vi "Pre Launch Init.vi"(11 "Tcp in":refnum<class "Tcp.lvclass">) -> (0 "error out":errorcluster, 3 "Tcp out":refnum<class "Tcp.lvclass">)   [LabVIEW 2022 SP3, in "Tcp.lvlib" / "Tcp.lvclass"]
doc: "(<B>Filename</B>: Actor Framework.lvlib:Actor.lvclass:Pre Launch Init.vi)\n\nDefines behavior that occurs after the Launch Actor method is invoked but before the actor's Actor Core method begins running.\n\nThe Pre Launch Init method is guaranteed to finish before the Launch Actor method returns to its caller and before the actor itself receives any messages. Any references that the Pre Launch Init method obtains are guaranteed to have the same lifetime as the actor itself. Any errors that the Pre Launch Init method returns will abort the launch.\n\nBy default, this method does nothing. A descendant class may override it to define behavior."
uses:
  Tcp.lvclass
  Tcp.lvclass/Tcp.ctl
  TcpSocket/Source/TcpSocket/TcpServer/TcpServer.lvclass
  <vilib>/ActorFramework/Actor/Actor.lvclass
  Tcp Messages/WaitForConnection Msg/WaitForConnection Msg.lvclass
  Logger/Source/Logger/_Level.ctl
  Logger/Source/Logger/Logger.lvclass
  DateTime/Source/DateTime.lvlib
  Logger/Source/Handler/Handler.lvclass
  Logger/Source/FileHandler/FileHandler.lvclass
  C:/Users/jakub/repos/gh/lv-cli-framework/Logger/Source/Handler/Handler.lvclass
  C:/Program Files (x86)/National Instruments/LabVIEW 2022/vi.lib/ActorFramework/Actor/Actor.lvclass
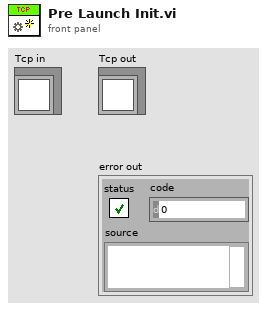
[diagram p1: front panel]
types:
  T1 = typedef "Logger.lvlib/Logger.lvclass/_Level.ctl" = enum16{"NOTSET", "DEBUG", "INFO", "WARNING", "ERROR", "CRITICAL"}
  T2 = enum16{"Standard", "Buffered", "CRLF", "Immediate"}
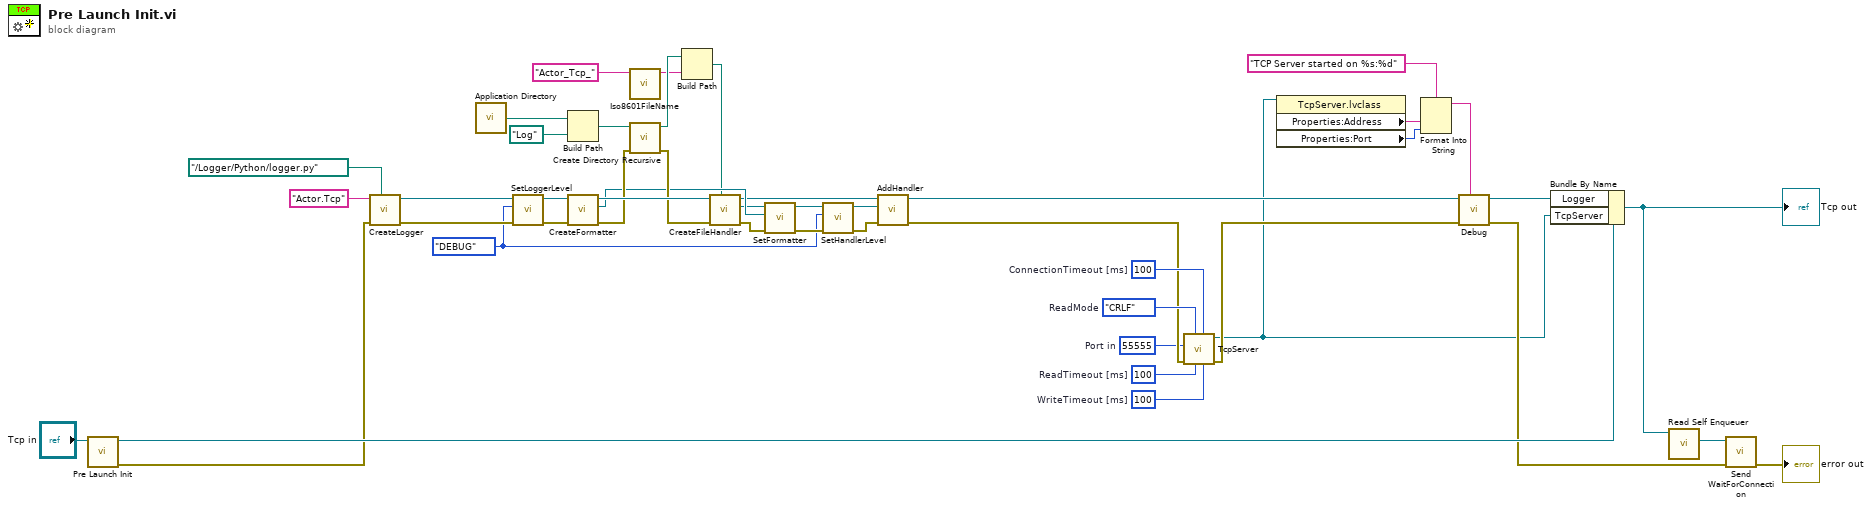
[diagram p0: block diagram]
diagram:
  w2 = _Level."DEBUG" ("Level")
  w43 = 100  # ConnectionTimeout [ms]
  w44 = 100  # WriteTimeout [ms]
  w45 = 100  # ReadTimeout [ms]
  w46 = T2."CRLF"  # ReadMode
  w16 = u16 55555  # Port in
  n1 = call-parent "Pre Launch Init.vi"("Actor in"="Tcp in") -> ("error out"=w23:errorcluster, "Actor out"=w42:refnum<class "Tcp.lvclass">)  [unwired: 9 in]
  n2 = call "CreateLogger.vi"("ModulePath"=path "../Logger/Python/logger.py" ("name or relative path"), "error in (no error)"=w23, "Name"="Actor.Tcp") -> ("error out"=w38:errorcluster, "Logger"=w37:refnum<class "Logger.lvclass">)  [unwired: 7 in]
  n3 = call <vilib>:"Application Directory.vi"() -> ("Application Directory"=w9:path)
  n4 = call-dynamic "SetLoggerLevel.vi"("error in (no error)"=w38, "Level"=w2, "Logger in"=w37) -> ("error out"=w35:errorcluster, "Logger out"=w36:refnum<class "Logger.lvclass">)  [unwired: 7 in]
  n5 = Build Path(base path=w9, name or relative path=path "Log") -> (appended path=w7:path)
  n6 = call-dynamic "CreateFormatter.vi"("error in (no error)"=w35, "Logger in"=w36) -> ("error out"=w32:errorcluster, "Formatter"=w28:refnum<class "Formatter.lvclass">, "Logger out"=w34:refnum<class "Logger.lvclass">)  [unwired: 7 in]
  n7 = call "Iso8601FileName.vi"("Prefix ('')"="Actor_Tcp_") -> ("FileName"=w5:string)  [unwired: 10 in]
  n8 = call <vilib>:"Create Directory Recursive.vi"("error in (no error)"=w32, "directory"=w7) -> ("error out"=w31:errorcluster, "directory copy"=w6:path)  [unwired: 3 in, 1 out]
  n9 = Build Path(base path=w6, name or relative path=w5) -> (appended path=w4:path)
  n10 = call-dynamic "CreateFileHandler.vi"("FIlePath"=w4, "error in (no error)"=w31, "Logger in"=w34) -> ("error out"=w30:errorcluster, "FileHandler"=w27:refnum<class "FileHandler.lvclass">, "Logger out"=w3:refnum<class "Logger.lvclass">)  [unwired: 6 in]
  n11 = call "SetFormatter.vi"("error in (no error)"=w30, "Formatter in"=w28, "Handler in"=w27) -> ("error out"=w29:errorcluster, "Handler out"=w26:refnum<class "FileHandler.lvclass">)  [unwired: 6 in, 1 out]
  n12 = call "SetHandlerLevel.vi"("error in (no error)"=w29, "Level"=w2, "Handler in"=w26) -> ("error out"=w25:errorcluster, "Handler out"=w24:refnum<class "Handler.lvclass">)  [unwired: 7 in]
  n13 = call-dynamic "AddHandler.vi"("error in (no error)"=w25, "Handler in"=w24, "Logger in"=w3) -> ("error out"=w22:errorcluster, "Logger out"=w19:refnum<class "Logger.lvclass">)  [unwired: 6 in, 1 out]
  n14 = call "TcpServer.vi"("WriteTimeout [ms] (5000)"=w44, "ConnectionTimeout [ms] (5000)"=w43, "ReadTimeout [ms] (5000)"=w45, "ReadMode (Standard)"=w46, "error in (no error)"=w22, "Port in (0)"=w16) -> ("error out"=w21:errorcluster, "TcpServer"=w15:refnum<class "TcpServer.lvclass">)  [unwired: 3 in, 1 out]
  n15 = property class="TcpServer.lvclass"(reference=w15) -> ("Properties:Address"=w14:string, "Properties:Port"=w13:u16)  [unwired: 1 in, 2 out]
  n16 = Format Into String(format string="TCP Server started on %s:%d", w14, w13) -> (resulting string=w12:string)  [unwired: 2 in, 1 out]
  n17 = call-dynamic "Debug.vi"("Message"=w12, "error in (no error)"=w21, "Logger in"=w19) -> ("error out"=w20:errorcluster, "Logger out"=w18:refnum<class "Logger.lvclass">)  [unwired: 7 in]
  n18 = Bundle By Name(cluster=w42, "Logger"=w18, "TcpServer"=w15) -> (w41:refnum<class "Tcp.lvclass">)
  "Tcp out" <- w41
  n19 = call <vilib>:"Read Self Enqueuer.vi"("Actor"=w41) -> ("Self Enqueuer"=w40:refnum<class "Message Enqueuer.lvclass">)  [unwired: 10 in]
  n20 = call "Send WaitForConnection.vi"("error in (no error)"=w20, "Message Enqueuer"=w40) -> ("error out"=→"error out":errorcluster)  [unwired: 8 in, 1 out]
